vi "OpenMultChannels.vi"(2 "error in (no error)":errorcluster, 3 "Channels to be opened":string="5102,5103,7103,7106") -> (0 "error out":errorcluster)   [LabVIEW 2012]
doc: "Open channels specified in comma-delimited list"
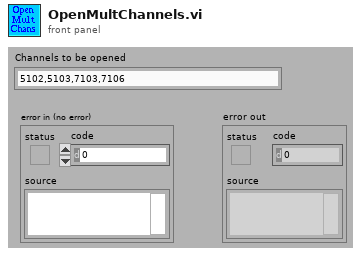
[diagram p1: front panel]
types:
  T1 = enum16{"N1911A", "Siggen", "34980a", "E4418B", "Rvp8"}
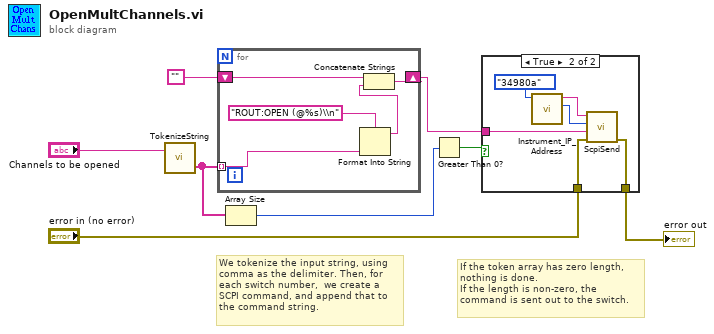
[diagram p0: block diagram]
diagram:
  # "If the token array has zero length, nothing is done.\nIf the length is non-zero, the command is sent out to the switch."
  # "We tokenize the input string, using comma as the delimiter. Then, for each switch number,  we create a SCPI command, and append that to the command string."
  n1 = call "TokenizeString.vi"("String to be tokenized"="Channels to be opened") -> ("Output array"=w2:string[])  [unwired: 2 in]
  n2 = for {
    tunnel: w2 -> [w12] mode=indexing
    shift-right: [w11] -> w5
    shift-left: "" -> [w10]
    n3 = Format Into String(format string="ROUT:OPEN (@%s)\\n", w12) -> (resulting string=w9:string)  [unwired: 2 in, 1 out]
    n4 = Concatenate Strings(w10, w9) -> (w11:string)
  }
  n5 = Array Size(array=w2) -> (size(s)=w1:i32)
  n6 = Greater Than 0?(x=w1) -> (x > 0?=w6:bool)
  n7 = case shown="True" w6 {
    tunnel: w5 -> [_ w20]
    tunnel: "error in (no error)" -> [w14 w19]
    tunnel: [w14 w18] -> w3
    frame False {
    }
    frame True {
      n8 = call "Instrument_IP_Address.vi"("Instrument"=T1."34980a") -> ("Port"=w16:u16, "IP Address"=w15:string)  [unwired: 9 in]
      n9 = call "ScpiSend.vi"("error in (no error)"=w19, "Command"=w20, "TCP port"=w16, "IP Address"=w15) -> ("error out"=w18:errorcluster)  [unwired: 7 in]
    }
  }
  "error out" <- w3
